vi "Folder_creation_calibration_04_03_2020.vi"() -> (2 "path":path, 3 "date/time string":string, 4 "calibration log":path)   [LabVIEW 2015]
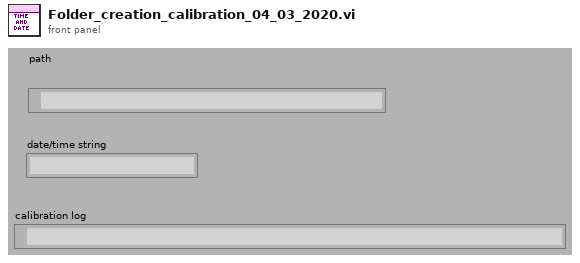
[diagram p1: front panel]
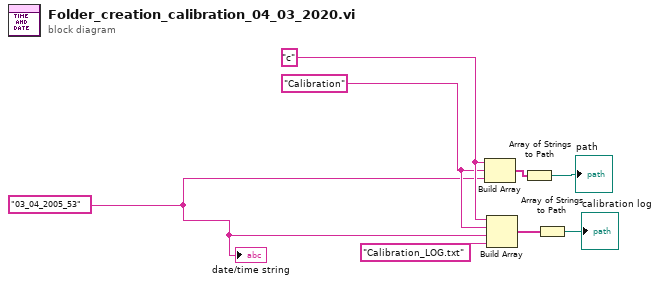
[diagram p0: block diagram]
diagram:
  w1 = "03_04_2005_53" ("date/time string")
  w5 = "Calibration" ("element")
  w6 = "c"
  n1 = Build Array(w6, w5, w1) -> (w8:string[])
  n2 = Build Array(w6, w5, w1, "Calibration_LOG.txt" ("element")) -> (w3:string[])
  n3 = Array of Strings to Path(0:w8) -> (2:→"path":path)  [unwired: 1 out]
  n4 = Array of Strings to Path(0:w3) -> (2:→"calibration log":path)  [unwired: 1 out]
  "date/time string" <- w1
